vi "Test JKI SM Helper.vi"() -> ()   [LabVIEW 2013]
uses:
  source/JKI State Machine API/source/JKI SM/JKI SM.lvclass/JKI SM.ctl
  source/JKI State Machine API/source/JKI SM/JKI SM.lvclass
  source/JKI State Machine API/tests/TEST JKI State Machine API.lvlib
panel:
  out "error out":errorcluster
  in  "EventStructure?":bool
  # "Run this VI to lauch the JKI State Machine helper on a template VI"
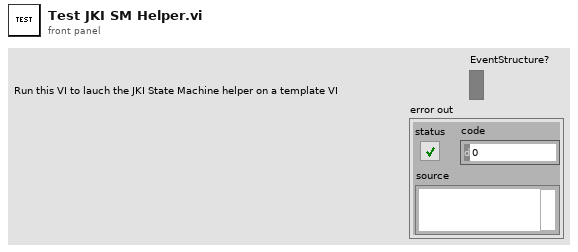
[diagram p1: front panel]
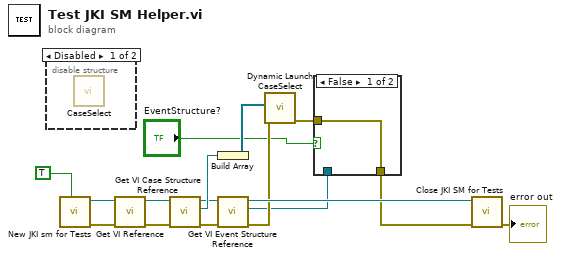
[diagram p0: block diagram]
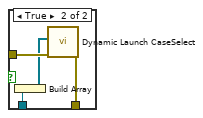
[diagram p3: hidden frame]
diagram:
  n1 = disable-structure shown="Disabled" {
    frame Disabled {
      n2 = call "CaseSelect.vi"() -> ()  [unwired: 12 in]
    }
    frame Enabled {
    }
  }
  n3 = call "New JKI sm for Tests.vi"("Open SM FP (for debugging)"=TRUE) -> ("error out"=w15:errorcluster, "JKI SM out"=w16:refnum<class "JKI SM.lvclass">)  [unwired: 9 in]
  n4 = call "Get VI Reference.vi"("error in (no error)"=w15, "JKI SM in"=w16) -> ("error out"=w12:errorcluster, "JKI SM out"=w14:refnum<class "JKI SM.lvclass">)  [unwired: 7 in, 1 out]
  n5 = call "Get VI Case Structure Reference.vi"("error in (no error)"=w12, "JKI SM in"=w14) -> ("error out"=w8:errorcluster, "Case Structure ref"=w13:refnum<vi>, "JKI SM out"=w9:refnum<class "JKI SM.lvclass">)  [unwired: 7 in]
  n6 = Build Array(w13) -> (w10:refnum<vi>[])
  n7 = call "Get VI Event Structure Reference.vi"("error in (no error)"=w8, "JKI SM in"=w9) -> ("error out"=w6:errorcluster, "Event Structure ref"=w3:refnum<vi>, "JKI SM out"=w7:refnum<class "JKI SM.lvclass">)  [unwired: 7 in]
  n8 = call "Dynamic Launch CaseSelect.vi"("error in (no error)"=w6, "Active VI Sel. List[]"=w10) -> ("error out"=w5:errorcluster)  [unwired: 9 in]
  n9 = case shown="False" "EventStructure?" {
    tunnel: w5 -> [w17 w21]
    tunnel: [w17 w20] -> w4
    tunnel: w3 -> [_ w19]
    frame False {
    }
    frame True {
      n10 = Build Array(w19) -> (w18:refnum<vi>[])
      n11 = call "Dynamic Launch CaseSelect.vi"("error in (no error)"=w21, "Active VI Sel. List[]"=w18) -> ("error out"=w20:errorcluster)  [unwired: 9 in]
    }
  }
  n12 = call "Close JKI SM for Tests.vi"("error in (no error)"=w4, "JKI SM in"=w7) -> ("error out"=→"error out":errorcluster)  [unwired: 9 in]
